vi "Set Offset Voltage.vi"(8 "error in (no error)":errorcluster, 10 "Offset":dbl format="%.2f", 11 "VISA resource name":refnum<visa-resource-name>) -> (0 "error out":errorcluster, 3 "VISA resource name out":refnum<visa-resource-name>)   [LabVIEW 2020, in "Associated Research 78XX Series.lvlib"]
doc: "EO < value > - Edit the offset value"
uses:
  <instrlib>/Associated Research 78XX Series/Associated Research 78XX Series.lvlib
panel:
  out "concatenated string":string
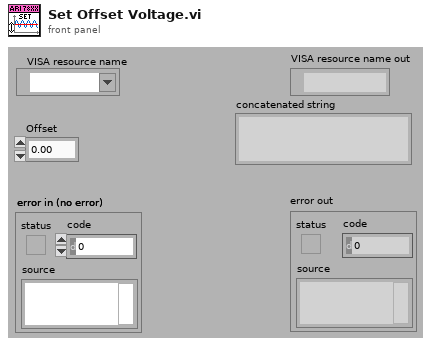
[diagram p1: front panel]
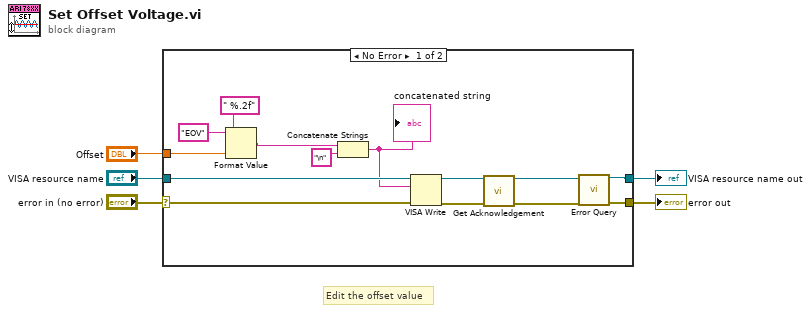
[diagram p0: block diagram]
diagram:
  # "Edit the offset value"
  n1 = case shown="No Error" "error in (no error)" {
    selector: "error in (no error)" -> [w15 w21]
    tunnel: [w12 w21] -> w4
    tunnel: [w11 w20] -> w2
    tunnel: "VISA resource name" -> [w19 w20]
    tunnel: "Offset" -> [w17 _]
    frame No Error {
      n2 = Format Value(string ("")="EOV", format string=" %.2f", value (0)=w17) -> (output string=w10:string)
      n3 = Concatenate Strings(w10, "\n" ("string")) -> (w13:string)
      "concatenated string" <- w13
      n4 = VISA Write(VISA resource name=w19, write buffer=w13, error in (no error)=w15) -> (VISA resource name out=w9:refnum<visa-resource-name>, error out=w7:errorcluster)  [unwired: 1 out]
      n5 = call <instrlib>:"Get Acknowledgement.vi"("VISA resource name"=w9, "error in (no error)"=w7) -> ("VISA resource name out"=w8:refnum<visa-resource-name>, "error out"=w6:errorcluster)  [unwired: 12 in]
      n6 = call <instrlib>:"Error Query.vi"("VISA resource name"=w8, "error in (no error)"=w6) -> ("VISA resource name out"=w11:refnum<visa-resource-name>, "error out"=w12:errorcluster)  [unwired: 10 in, 2 out]
    }
    frame Error {
    }
  }
  "error out" <- w4
  "VISA resource name out" <- w2
